vi "Initialize.vi"(8 "error in (no error)":errorcluster, 11 "AM in":refnum<class "AM.lvclass">) -> (0 "error out":errorcluster, 3 "AM out":refnum<class "AM.lvclass">)   [LabVIEW 2015, in "AM.lvclass"]
uses:
  AM.lvclass
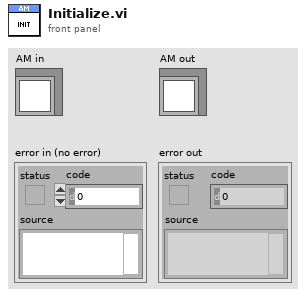
[diagram p1: front panel]
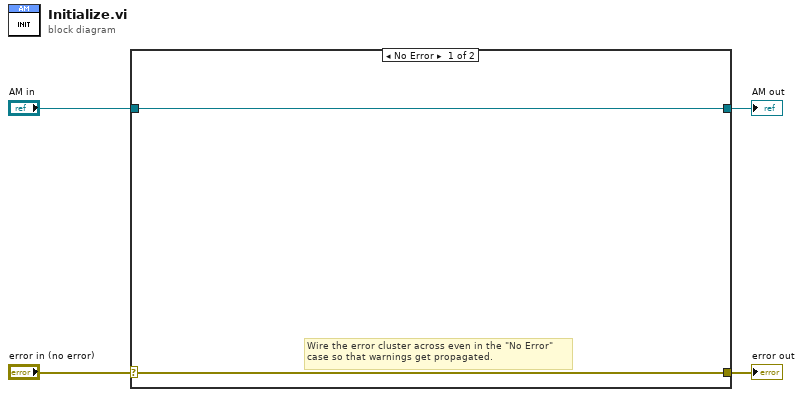
[diagram p0: block diagram]
diagram:
  n1 = case shown="No Error" "error in (no error)" {
    selector: "error in (no error)" -> [w5 w8]
    tunnel: [w5 w8] -> w3
    tunnel: [w6 w7] -> w1
    tunnel: "AM in" -> [w6 w7]
    frame No Error {
      # "Wire the error cluster across even in the \"No Error\"\ncase so that warnings get propagated."
    }
    frame Error {
    }
  }
  "error out" <- w3
  "AM out" <- w1
